vi "serial_port_setup.vi"(5 "baud rate (9600)":u32=9600 caption="波特率(9600)", 6 "flow control (0:none)":u16(ring) caption="流控制（0:无）" items=["无", "XON/XOFF", "RTS/CTS", "XON/XOFF & RTS/CTS", "DTR/DSR", "XON/XOFF & DTR/DSR"], 7 "data bits (8)":u16=8 caption="数据比特(8)" min=5 max=8 step=1, 8 "错误输入（无错误）":errorcluster, 9 "stop bits (10: 1 bit)":u16(ring)=10 caption="停止位（10: 1位）" items=["1.0"=10, "1.5"=15, "2.0"=20], 10 "parity (0:none)":enum16{"None", "Odd", "Even", "Mark", "Space"}(ring) caption="奇偶（0:无）", 11 "VISA引用句柄输入":refnum<visa-resource-name> caption="VISA资源名称") -> (0 "错误输出":errorcluster, 3 "VISA引用句柄输出":refnum<visa-resource-name> caption="VISA资源名称输出")   [LabVIEW 2014]
uses:
  <vilib>/Instr/_visa.llb/VISA Configure Serial Port (Instr).vi
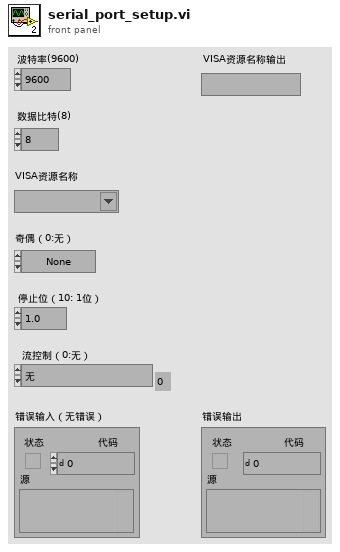
[diagram p1: front panel]
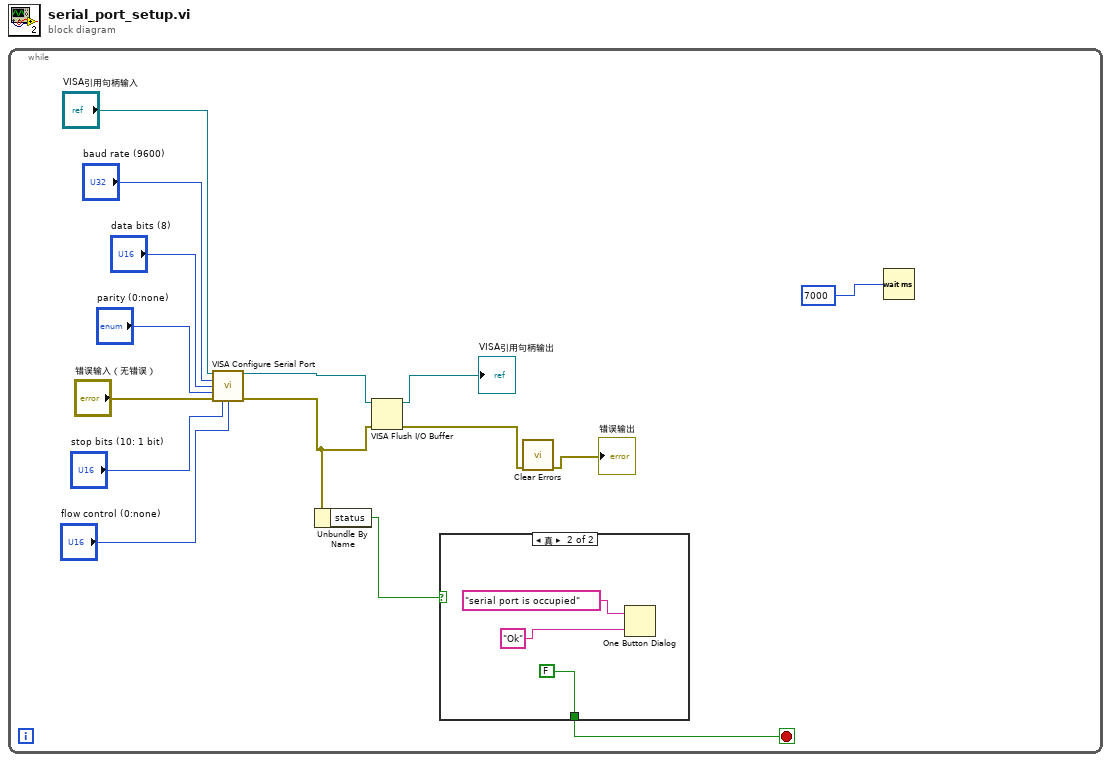
[diagram p0: block diagram]
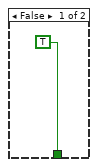
[diagram p2: hidden frame]
diagram:
  n1 = while {
    stop <- w2 stop-if-true
    n2 = call-poly "VISA Configure Serial Port"("VISA resource name"="VISA引用句柄输入", "baud rate (9600)"="baud rate (9600)", "data bits (8)"="data bits (8)", "parity (0:none)"="parity (0:none)", "error in (no error)"="错误输入（无错误）", "stop bits (10: 1 bit)"="stop bits (10: 1 bit)", "flow control (0:none)"="flow control (0:none)") -> ("VISA resource name out"=w10:refnum<visa-resource-name>, "error out"=w12:errorcluster)  [unwired: 7 in]
    n3 = Unbundle By Name(w12) -> ("status"=w13:bool)
    n4 = VISA Flush I/O Buffer(VISA resource name=w10, error in (no error)=w12) -> (VISA resource name out=→"VISA引用句柄输出":refnum<visa-resource-name>, error out=w15:errorcluster)  [unwired: 1 in]
    n5 = case shown="真" w13 {
      tunnel: [TRUE FALSE] -> w2
      frame False {
      }
      frame True {
        n6 = One Button Dialog(message="serial port is occupied", button name ("OK")="Ok") -> ()  [unwired: 1 out]
      }
    }
    n7 = call <vilib>:"Clear Errors.vi"("error in (no error)"=w15) -> ("error out"=→"错误输出":errorcluster)  [unwired: 5 in, 1 out]
    n8 = Wait (ms)(milliseconds to wait=u32 7000 ("等待时间（毫秒）")) -> ()  [unwired: 1 out]
  }
